vi "ATM_FP.ScanFP.PopUp.vi"(6 "debug?":bool=TRUE, 7 "machineLog":refnum<vi>, 8 "errorIn":errorcluster, 11 "VISA":refnum<visa-resource-name>) -> (0 "errorOut":errorcluster, 2 "fpID":u16, 3 "fpFound":bool)   [LabVIEW 2020]
uses:
  __ATM__FP__SCAN__FP__STATE__.ctl
  __ATM__FP__COMMUNICATION__COMMAND__.ctl
panel:
  in  "Cancel Button":bool
  out "Scan ID":string
  in  "machineLog":string
  in  "userMsg":string
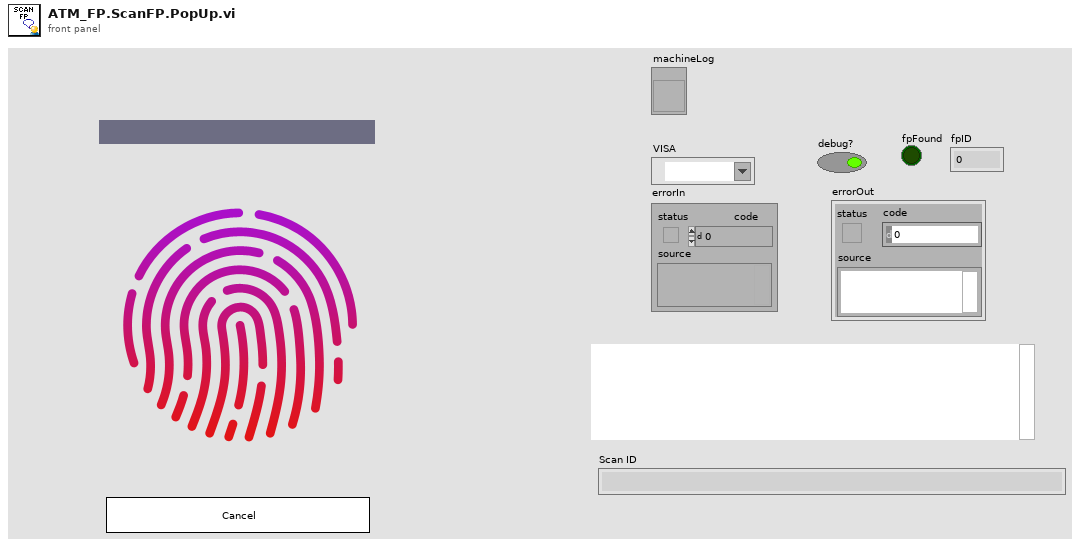
[diagram p1: front panel]
types:
  T1 = cluster{"VISA":refnum<visa-resource-name>, "userMsg":refnum<vi>, "machineLog":refnum<vi>, "openVisa?":bool, "fpFound":bool, "fpID":u16}
  T2 = typedef "__ATM__FP__SCAN__FP__STATE__.ctl" = enum16{"Init", "Scan FP", "Generate  FP to store to CharBuffer", "Search FP from FP Database", "Fail to scan", "Add -- Scan FP 1st", "Add -- Generate  FP to store to CharBuffer 1", "Add -- Scan FP 2nd", "Add -- Generate  FP to store to CharBuffer 2", "Add -- Register and create FP template", "Add -- Store FP template in FP database", "End"}
  T3 = typedef "__ATM__FP__COMMUNICATION__COMMAND__.ctl" = enum16{"1. PS_GetImage -- Detect FP Image", "2. PS_GenChar -- Generate FP Template from Image [BufferChar1]", "2. PS_GenChar -- Generate FP Template from Image [BufferChar2]", "3. PS_Match -- Compare 2 FP Template", "4. PS_Search -- Search fingerprint", "5. PS_RegModel -- Generate template", "6. PS_StoreChar -- Store template", "7. PS_LoadChar -- FP Database -->Feature Buffer", "8. PS_UpChar --  Upload Feature Buff --> PC", "12. PS_DeletChar -- Delete template", "13. PS_Empty -- Delete all FP templates", "15. S_ReadSysPara -- Read system basic parameters"}
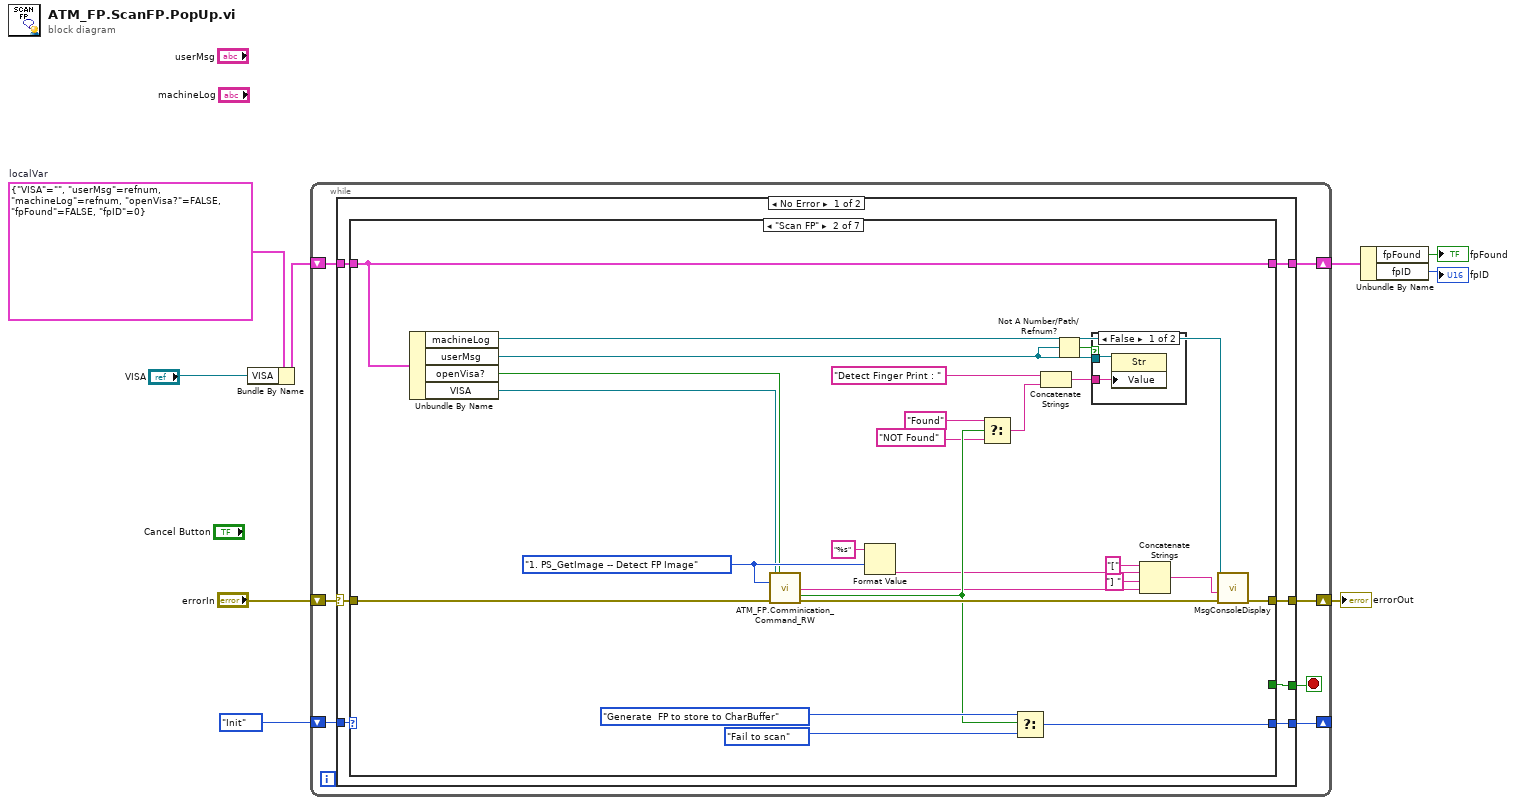
[diagram p0: block diagram]
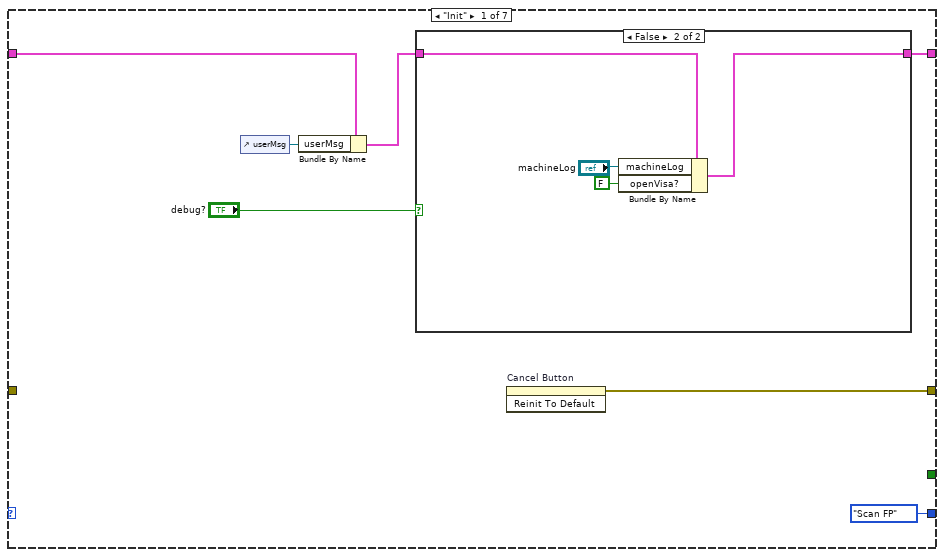
[diagram p2: hidden frame]
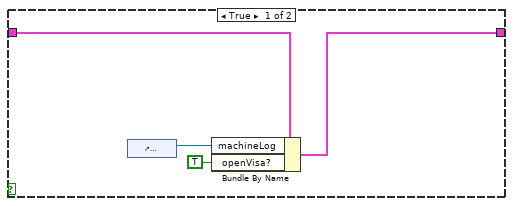
[diagram p3: hidden frame]
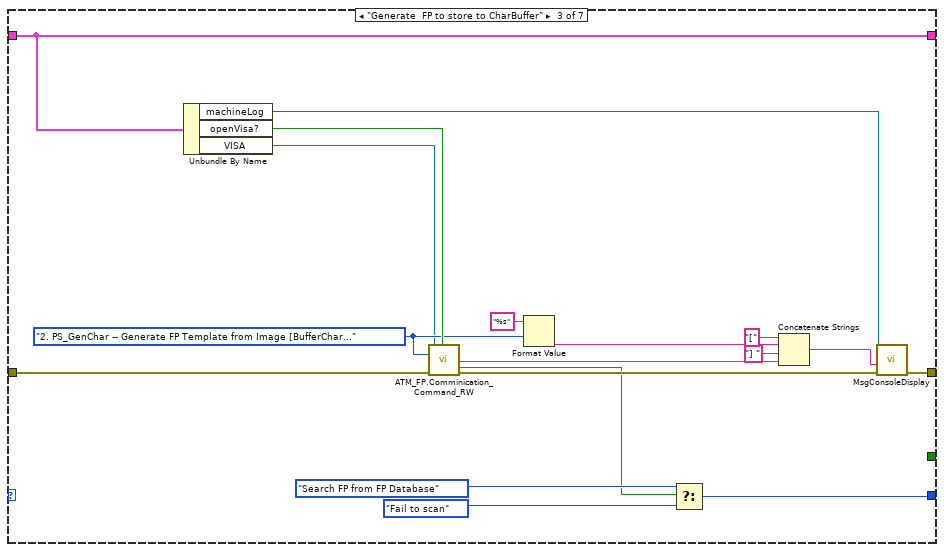
[diagram p5: hidden frame]
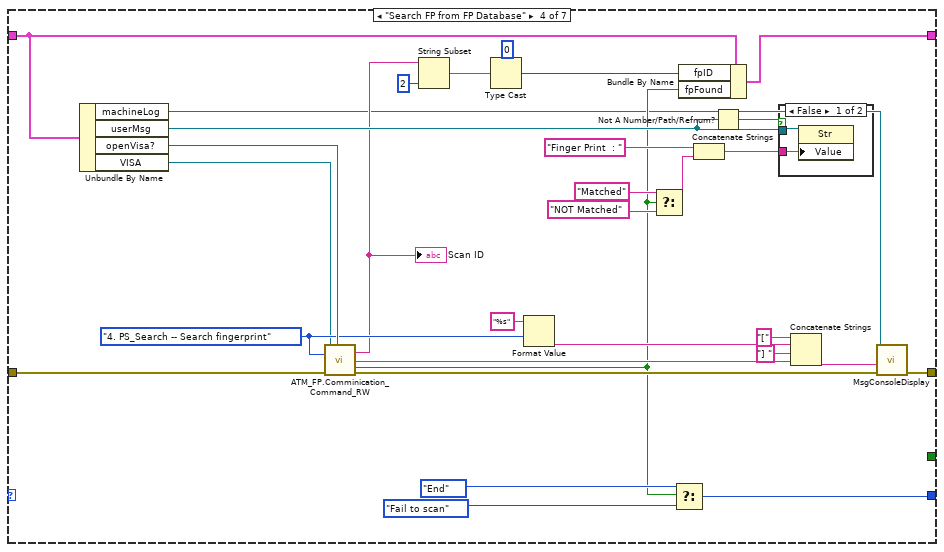
[diagram p6: hidden frame]
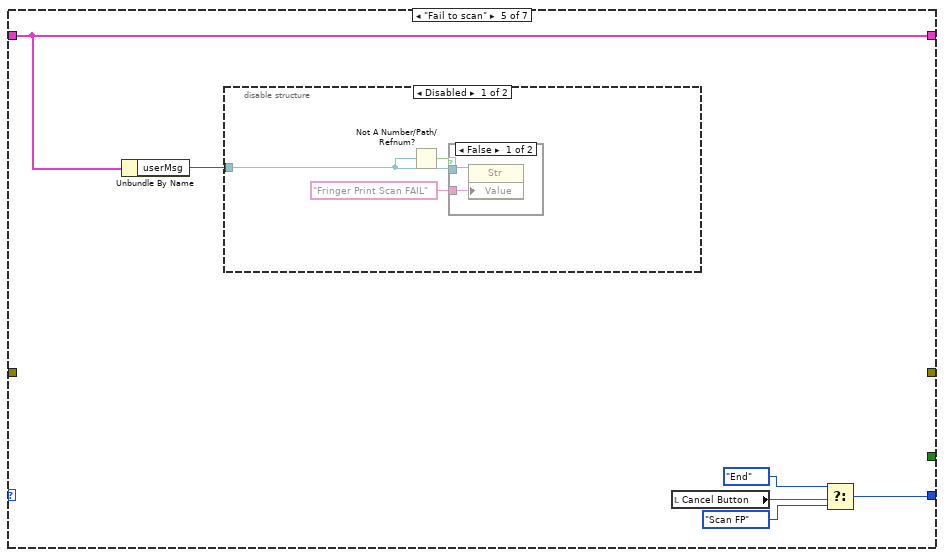
[diagram p8: hidden frame]
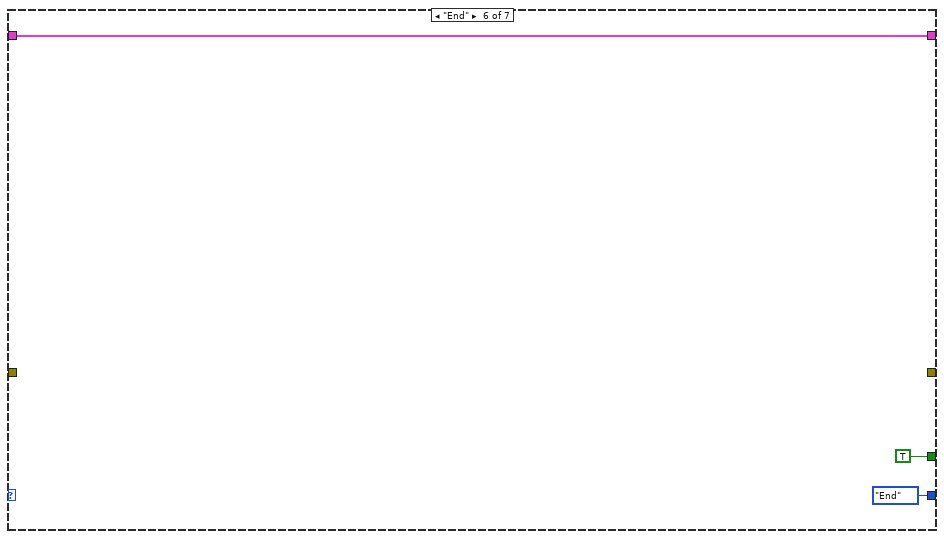
[diagram p11: hidden frame]
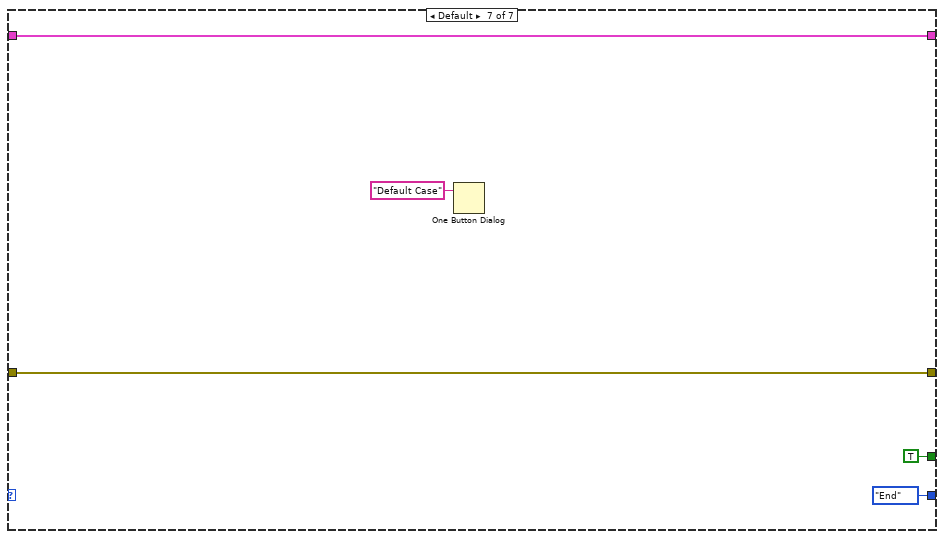
[diagram p12: hidden frame]
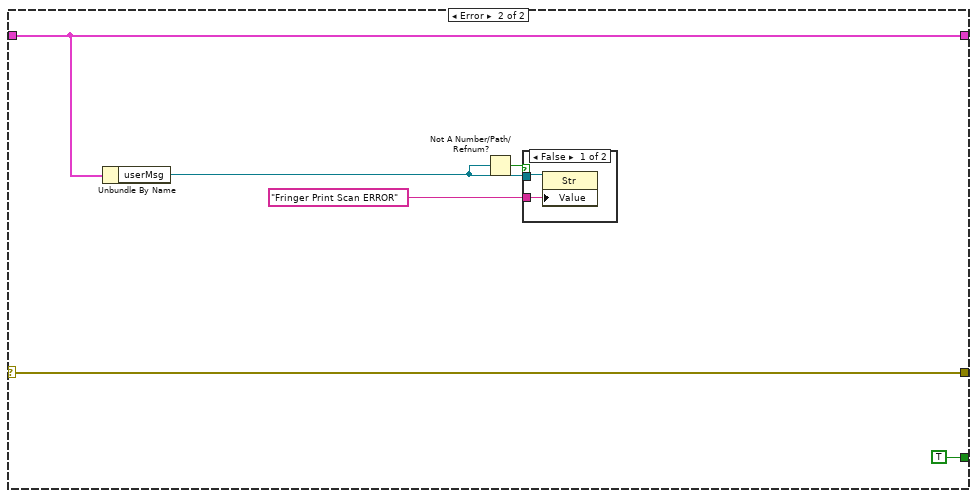
[diagram p13: hidden frame]
diagram:
  w7 = T1 {"VISA"="", "userMsg"=refnum, "machineLog"=refnum, "openVisa?"=FALSE, "fpFound"=FALSE, "fpID"=0}  # localVar
  n1 = Bundle By Name(cluster=w7, "VISA"="VISA") -> (w6:T1)
  n2 = while {
    shift-right: [w15] -> w4
    shift-left: "errorIn" -> [w16]
    shift-right: [w13] -> _
    shift-left: __ATM__FP__SCAN__FP__STATE__."Init" -> [w14]
    shift-right: [w11] -> w3
    shift-left: w6 -> [w12]
    stop <- w10 stop-if-true
    n3 = case shown="No Error" w16 {
      selector: w16 -> [w23 w141]
      tunnel: [w22 w141] -> w15
      tunnel: w14 -> [w21 _]
      tunnel: [w20 _] -> w13
      tunnel: w12 -> [w19 w136]
      tunnel: [w18 w136] -> w11
      tunnel: [w17 TRUE] -> w10
      frame No Error {
        n4 = case shown="\"Scan FP\"" w21 {
          tunnel: w23 -> [_ w63 w83 w114 _ _ w134]
          tunnel: [w27 w58 w78 w109 _ _ w134] -> w22
          tunnel: [__ATM__FP__SCAN__FP__STATE__."Scan FP" w61 w81 w112 w117 __ATM__FP__SCAN__FP__STATE__."End" __ATM__FP__SCAN__FP__STATE__."End"] -> w20
          tunnel: w19 -> [w26 w57 w77 w93 w121 w130 w135]
          tunnel: [w29 w57 w77 w92 w121 w130 w135] -> w18
          tunnel: [_ _ _ _ _ TRUE TRUE] -> w17
          frame "Init" {
            n5 = control-ref of="userMsg"() -> (w24:refnum<vi>)
            n6 = Bundle By Name(cluster=w26, "userMsg"=w24) -> (w25:T1)
            n7 = case shown="False" "debug?" {
              tunnel: w25 -> [w34 w38]
              tunnel: [w33 w37] -> w29
              frame True {
                n8 = control-ref of="machineLog"() -> (w32:refnum<vi>)
                n9 = Bundle By Name(cluster=w34, "machineLog"=w32, "openVisa?"=TRUE ("debug?")) -> (w33:T1)
              }
              frame False {
                n10 = Bundle By Name(cluster=w38, "machineLog"="machineLog", "openVisa?"=FALSE ("debug?")) -> (w37:T1)
              }
            }
            n11 = invoke on="Cancel Button" class="Bool (strict)" method="Reinit To Default"() -> (error out=w27:errorcluster)  [unwired: 3 in, 2 out]
          }
          frame "Scan FP" {
            w47 = __ATM__FP__COMMUNICATION__COMMAND__."1. PS_GetImage -- Detect FP Image" ("Command")
            n12 = Unbundle By Name(w57) -> ("machineLog"=w39:refnum<vi>, "userMsg"=w56:refnum<vi>, "openVisa?"=w41:bool, "VISA"=w42:refnum<visa-resource-name>)
            n13 = call "ATM_FP.Comminication_Command_RW.vi"("VISA"=w42, "openPort?"=w41, "Command"=w47, "error in (no error)"=w63) -> ("reponseOK?"=w54:bool, "confirmationMsg"=w48:string, "error IO"=w59:errorcluster)  [unwired: 5 in, 4 out]
            n14 = Format Value(format string="%s", value (0)=w47) -> (output string=w45:string)  [unwired: 1 in]
            n15 = Select(t="Found", s=w54, f="NOT Found") -> (s? t:f=w50:string)
            n16 = Select(t=__ATM__FP__SCAN__FP__STATE__."Generate  FP to store to CharBuffer", s=w54, f=__ATM__FP__SCAN__FP__STATE__."Fail to scan") -> (s? t:f=w61:T2)
            n17 = Concatenate Strings("Detect Finger Print : ", w50) -> (w49:string)
            n18 = Not A Number/Path/Refnum?(number/path/refnum=w56) -> (NaN/Path/Refnum?=w55:bool)
            n19 = case shown="False" w55 {
              tunnel: w56 -> [w65 _]
              tunnel: w49 -> [w64 _]
              frame False {
                n20 = property class="Str"(reference=w65, "Value"=w64) -> ()  [unwired: 1 in, 2 out]
              }
              frame True {
              }
            }
            n21 = Concatenate Strings("[", w45, "] " ("string"), w48) -> (w40:string)
            n22 = call <userlib>:"MsgConsoleDisplay.vi"("error in"=w59, "String For Write"=w40, "dialogIn"=w39) -> ("error out"=w58:errorcluster)  [unwired: 7 in, 1 out]
          }
          frame "Generate  FP to store to CharBuffer" {
            w73 = __ATM__FP__COMMUNICATION__COMMAND__."2. PS_GenChar -- Generate FP Template from Image [BufferChar1]" ("Command")
            n23 = Unbundle By Name(w77) -> ("machineLog"=w66:refnum<vi>, "openVisa?"=w76:bool, "VISA"=w68:refnum<visa-resource-name>)
            n24 = call "ATM_FP.Comminication_Command_RW.vi"("VISA"=w68, "openPort?"=w76, "Command"=w73, "error in (no error)"=w83) -> ("reponseOK?"=w75:bool, "confirmationMsg"=w74:string, "error IO"=w79:errorcluster)  [unwired: 5 in, 4 out]
            n25 = Format Value(format string="%s", value (0)=w73) -> (output string=w71:string)  [unwired: 1 in]
            n26 = Select(t=__ATM__FP__SCAN__FP__STATE__."Search FP from FP Database", s=w75, f=__ATM__FP__SCAN__FP__STATE__."Fail to scan") -> (s? t:f=w81:T2)
            n27 = Concatenate Strings("[", w71, "] " ("string"), w74) -> (w67:string)
            n28 = call <userlib>:"MsgConsoleDisplay.vi"("error in"=w79, "String For Write"=w67, "dialogIn"=w66) -> ("error out"=w78:errorcluster)  [unwired: 7 in, 1 out]
          }
          frame "Search FP from FP Database" {
            w99 = __ATM__FP__COMMUNICATION__COMMAND__."4. PS_Search -- Search fingerprint" ("Command")
            n29 = Unbundle By Name(w93) -> ("machineLog"=w84:refnum<vi>, "userMsg"=w108:refnum<vi>, "openVisa?"=w106:bool, "VISA"=w94:refnum<visa-resource-name>)
            n30 = call "ATM_FP.Comminication_Command_RW.vi"("VISA"=w94, "openPort?"=w106, "Command"=w99, "error in (no error)"=w114) -> ("returnParameter"=w90:string, "reponseOK?"=w91:bool, "confirmationMsg"=w100:string, "error IO"=w110:errorcluster)  [unwired: 5 in, 3 out]
            "Scan ID" <- w90
            n31 = String Subset(string=w90, length (rest)=2 ("length (rest)")) -> (substring=w88:string)  [unwired: 1 in]
            n32 = Type Cast(type=u16 0, x=w88) -> (*(type *) &x=w86:u16)
            n33 = Format Value(format string="%s", value (0)=w99) -> (output string=w97:string)  [unwired: 1 in]
            n34 = Select(t="Matched", s=w91, f="NOT Matched") -> (s? t:f=w102:string)
            n35 = Select(t=__ATM__FP__SCAN__FP__STATE__."End", s=w91, f=__ATM__FP__SCAN__FP__STATE__."Fail to scan") -> (s? t:f=w112:T2)
            n36 = Bundle By Name(cluster=w93, "fpID"=w86, "fpFound"=w91) -> (w92:T1)
            n37 = Concatenate Strings("Finger Print  : ", w102) -> (w101:string)
            n38 = Not A Number/Path/Refnum?(number/path/refnum=w108) -> (NaN/Path/Refnum?=w107:bool)
            n39 = case shown="False" w107 {
              tunnel: w108 -> [w116 _]
              tunnel: w101 -> [w115 _]
              frame False {
                n40 = property class="Str"(reference=w116, "Value"=w115) -> ()  [unwired: 1 in, 2 out]
              }
              frame True {
              }
            }
            n41 = Concatenate Strings("[", w97, "] " ("string"), w100) -> (w85:string)
            n42 = call <userlib>:"MsgConsoleDisplay.vi"("error in"=w110, "String For Write"=w85, "dialogIn"=w84) -> ("error out"=w109:errorcluster)  [unwired: 7 in, 1 out]
          }
          frame "Fail to scan" {
            n43 = Unbundle By Name(w121) -> ("userMsg"=w122:refnum<vi>)
            n44 = disable-structure shown="Disabled" {
              disable-tunnel: w122 -> [w125 _]
              frame Disabled {
                n45 = Not A Number/Path/Refnum?(number/path/refnum=w125) -> (NaN/Path/Refnum?=w124:bool)
                n46 = case shown="False" w124 {
                  tunnel: w125 -> [w127 _]
                  tunnel: "Fringer Print Scan FAIL" -> [w126 _]
                  frame False {
                    n47 = property class="Str"(reference=w127, "Value"=w126) -> ()  [unwired: 1 in, 2 out]
                  }
                  frame True {
                  }
                }
              }
              frame Enabled {
              }
            }
            n48 = local read "Cancel Button"() -> (w120:bool)
            n49 = Select(t=__ATM__FP__SCAN__FP__STATE__."End", s=w120, f=__ATM__FP__SCAN__FP__STATE__."Scan FP") -> (s? t:f=w117:T2)
          }
          frame "End" {
          }
          frame Default {
            n50 = One Button Dialog(message="Default Case") -> ()  [unwired: 1 in, 1 out]
          }
        }
      }
      frame Error {
        n51 = Unbundle By Name(w136) -> ("userMsg"=w139:refnum<vi>)
        n52 = Not A Number/Path/Refnum?(number/path/refnum=w139) -> (NaN/Path/Refnum?=w138:bool)
        n53 = case shown="False" w138 {
          tunnel: w139 -> [w143 _]
          tunnel: "Fringer Print Scan ERROR" -> [w142 _]
          frame False {
            n54 = property class="Str"(reference=w143, "Value"=w142) -> ()  [unwired: 1 in, 2 out]
          }
          frame True {
          }
        }
      }
    }
  }
  "errorOut" <- w4
  n55 = Unbundle By Name(w3) -> ("fpFound"=→"fpFound":bool, "fpID"=→"fpID":u16)
